vi "KE_scan_Gaussian_Fit.vi"(7 "NI DAQ (t) / Keithley (f)":bool, 8 "GaussFit der (f, def) / raw (t)":bool, 9 "Channel":i32=1 min=0 max=7 step=1, 10 "div I zero":bool=TRUE, 11 "KE scan Array":dbl[][](array[numeric])) -> (0 "error out":errorcluster, 1 "center":dbl format="%.1f", 2 "FWHM":dbl format="%.1f", 3 "KE scan Array OUT":dbl[][](array[numeric]), 4 "residue":dbl, 5 "XY Graph Array":cluster{dbl[], "Best Gaussian Fit":dbl[]}[](array[cluster]), 6 "offset":dbl)   [LabVIEW 2018]
uses:
  <vilib>/Analysis/6fits.llb/Curve Fitting Criteria.ctl
  <vilib>/Utility/file.llb/Read From Spreadsheet File (DBL).vi
  <vilib>/Analysis/NI_AALPro.lvlib
panel:
  out "XY Graph":T1(graph)
  in  "Density Factor (5)":dbl=5.0 format="%#_13g"
  out "Interpolated x-Axis":dbl[](array[numeric])
  in  "method (least square)":T2 items=["Least Square", "Least Absolute Residual", "Bisquare"]
  out "amplitude":dbl
  out "x-Axis":dbl[](array[numeric])
  out "abs(Derivative)":dbl[](array[numeric])
  out "Signal":dbl[](array[numeric])
  out "Best Gaussian Fit":dbl[](array[numeric])
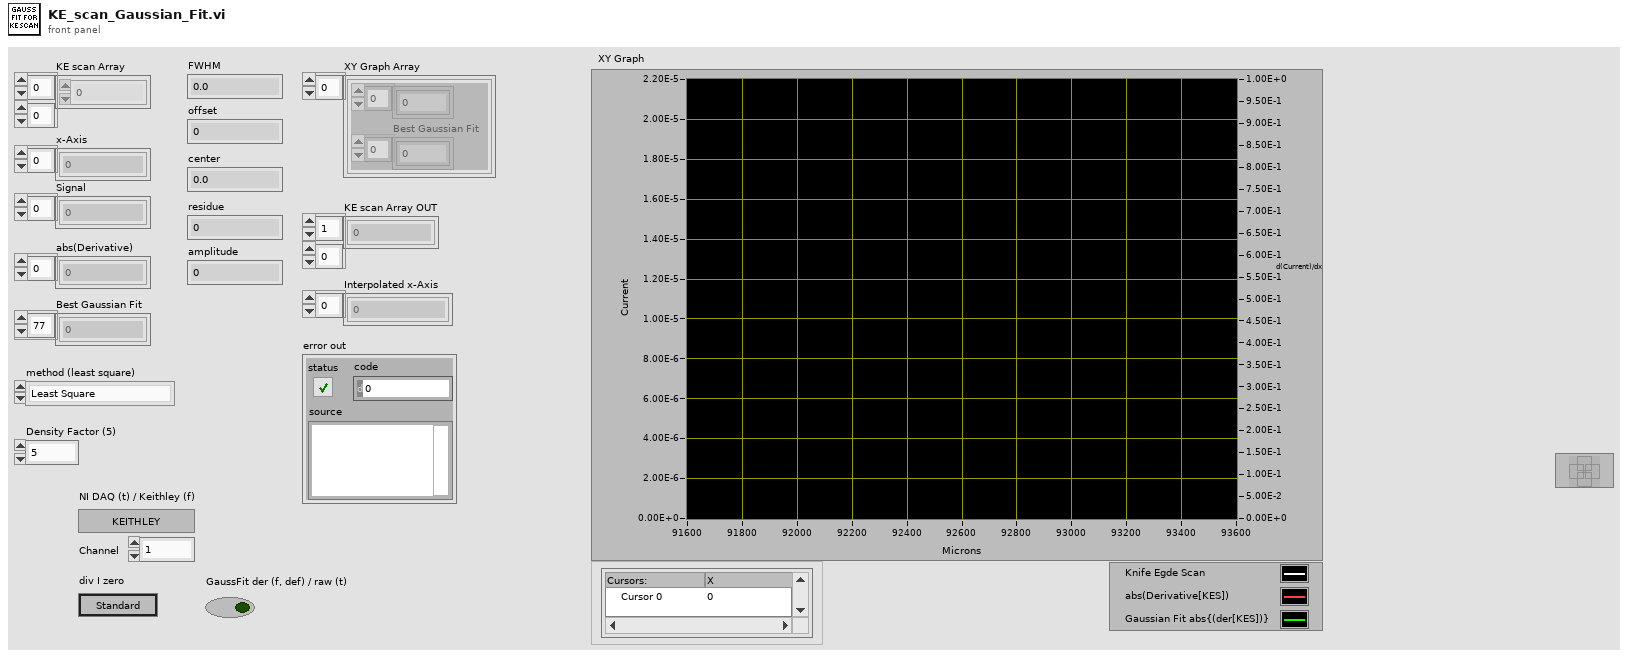
[diagram p1: front panel]
types:
  T1 = cluster{"Interpolated Array":dbl[], "Gaussian (Y)":dbl[]}[]
  T2 = typedef "NI_AALPro.lvlib/Curve Fitting Criteria.ctl" = u16
  T3 = cluster{"amp min":dbl, "amp max":dbl, "center min":dbl, "center max":dbl, "deviation min":dbl, "deviation max":dbl, "offset min":dbl, "offset max":dbl}
  T4 = cluster{"initial amplitude":dbl, "initial center":dbl, "initial standard deviation":dbl, "offset":dbl}
  T5 = cluster{"Interpolated Array":dbl[], "Gaussian (Y)":dbl[]}
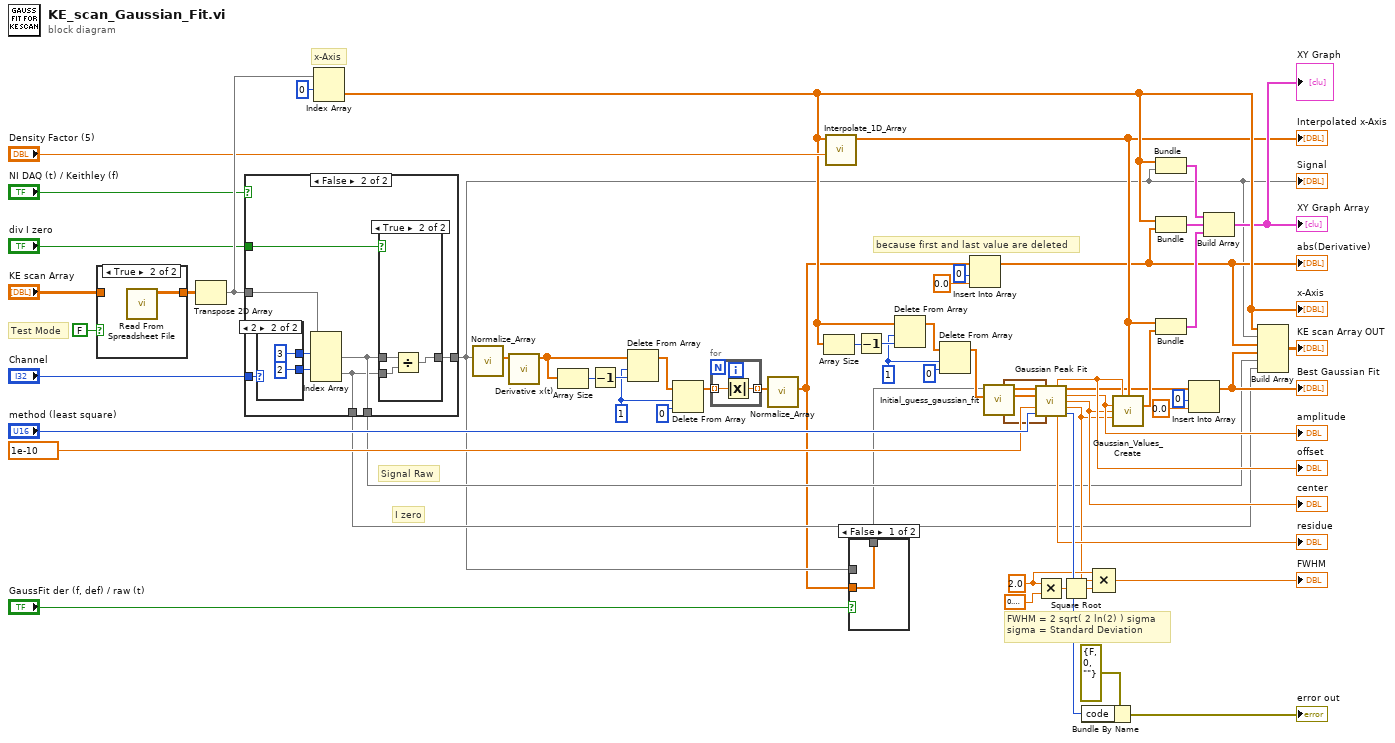
[diagram p0: block diagram]
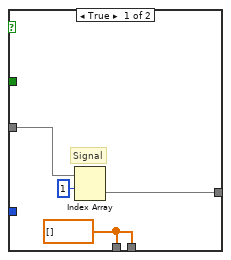
[diagram p3: hidden frame]
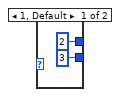
[diagram p5: hidden frame]
diagram:
  w40 = 1 ("length")
  w51 = 2.0 ("x")
  w59 = 1 ("length")
  # "I zero"
  # "Signal Raw"
  # "because first and last value are deleted"
  # "Test Mode"
  # "x-Axis"
  # "FWHM = 2 sqrt( 2 ln(2) ) sigma\nsigma = Standard Deviation"
  n1 = case shown="True" FALSE {
    tunnel: "KE scan Array" -> [w65 _]
    tunnel: [w65 w66] -> w27
    frame False {
    }
    frame True {
      n2 = call-poly <vilib>:"Read From Spreadsheet File.vi"() -> ("all rows"=w66:dbl[][])  [unwired: 7 in, 4 out]
    }
  }
  n3 = Transpose 2D Array(2D array=w27) -> (transposed array=w63:dbl[][])
  n4 = case shown="False" "NI DAQ (t) / Keithley (f)" {
    tunnel: w63 -> [w69 w77]
    tunnel: [w68 w74] -> w4
    tunnel: "Channel" -> [_ w75]
    tunnel: "div I zero" -> [_ w73]
    tunnel: [w67 w72] -> w6
    tunnel: [w67 w71] -> w5
    frame True {
      w67 = dbl[] []
      # "Signal"
      n5 = Index Array(array=w69, index (row)=1) -> (element=w68:dbl[])  [unwired: 1 in]
    }
    frame False {
      n6 = case shown="2" w75 {
        tunnel: [2 ("index (row)") 3 ("index (row)")] -> w78
        tunnel: [3 ("index (row)") 2 ("index (row)")] -> w76
        frame 1, Default {
        }
        frame 2 {
        }
      }
      n7 = Index Array(array=w77, index (row) #1=w78, index (row) #2=w76) -> (element #1=w72:dbl[], element #2=w71:dbl[])  [unwired: 2 in]
      n8 = case shown="True" w73 {
        tunnel: w72 -> [w79 w82]
        tunnel: w71 -> [_ w81]
        tunnel: [w79 w80] -> w74
        frame False {
        }
        frame True {
          n9 = Divide(x=w82, y=w81) -> (x/y=w80:dbl[])
        }
      }
    }
  }
  "Signal" <- w4
  n10 = Index Array(array=w63, index (row)=0) -> (element=w24:dbl[])  [unwired: 1 in]
  "x-Axis" <- w24
  n11 = call "Normalize_Array.vi"("array"=w4) -> ("normalized array"=w34:dbl[])  [unwired: 10 in]
  n12 = call <vilib>:"Derivative x(t).vi"("X"=w34) -> ("dX/dt"=w47:dbl[])  [unwired: 9 in, 1 out]
  n13 = Array Size(array=w47) -> (size(s)=w62:i32)
  n14 = Decrement(x=w62) -> (x-1=w61:i32)
  n15 = Delete From Array(array=w47, length=w59, index=w61) -> (array with subset deleted=w60:dbl[])  [unwired: 1 out]
  n16 = Delete From Array(array=w60, length=w59, index=0) -> (array with subset deleted=w57:dbl[])  [unwired: 1 out]
  n17 = for {
    tunnel: w57 -> [w88] mode=indexing
    tunnel: [w87] -> w31 mode=indexing
    n18 = Absolute Value(x=w88) -> (abs(x)=w87:dbl)
  }
  n19 = call "Normalize_Array.vi"("array"=w31) -> ("normalized array"=w3:dbl[])  [unwired: 10 in]
  n20 = Array Size(array=w24) -> (size(s)=w43:i32)
  n21 = call "Interpolate_1D_Array.vi"("Density Factor"="Density Factor (5)", "x-Axis in"=w24) -> ("Interpolated Array"=w17:dbl[])  [unwired: 9 in]
  "Interpolated x-Axis" <- w17
  n22 = case shown="False" "GaussFit der (f, def) / raw (t)" {
    tunnel: w4 -> [_ w90]
    tunnel: w3 -> [w89 _]
    tunnel: [w89 w90] -> w2
    frame False {
    }
    frame True {
    }
  }
  n23 = Decrement(x=w43) -> (x-1=w42:i32)
  n24 = Delete From Array(array=w24, length=w40, index=w42) -> (array with subset deleted=w41:dbl[])  [unwired: 1 out]
  n25 = Delete From Array(array=w41, length=w40, index=0) -> (array with subset deleted=w46:dbl[])  [unwired: 1 out]
  n26 = Insert Into Array(array=w3, index=0, new element=0.0 ("new element/subarray")) -> (w15:dbl[])
  "abs(Derivative)" <- w15
  n27 = call "Initial_guess_gaussian_fit.vi"("x-Axis in"=w46, "Signal in"=w2) -> ("x-Axis out"=w45:dbl[], "Signal out"=w44:dbl[], "Parameter Bounds Cluster"=w26:T3, "Initial Guess Cluster"=w32:T4)  [unwired: 2 in, 4 out]
  n28 = call <vilib>:"Gaussian Peak Fit.vi"("Y"=w44, "initial guess"=w32, "X"=w45, "tolerance"=1e-10, "method"="method (least square)", "parameter bounds"=w26) -> ("offset"=w23:dbl, "Best Gaussian Fit"=w11:dbl[], "amplitude"=w22:dbl, "center"=w21:dbl, "standard deviation"=w20:dbl, "residue"=→"residue":dbl, "error"=w55:i32)  [unwired: 3 in]
  "center" <- w21
  "offset" <- w23
  "amplitude" <- w22
  n29 = Multiply(x=w51, y=0.6931471805599453) -> (x*y=w52:dbl)
  n30 = Square Root(x=w52) -> (sqrt(x)=w50:dbl)
  n31 = Bundle By Name(cluster=errorcluster {"status"=FALSE, "code"=0, "source"=""} ("error in"), "code"=w55) -> (→"error out":errorcluster)
  n32 = Compound Arithmetic op=MULTIPLY(w51, w20, w50) -> (→"FWHM":dbl)
  n33 = call "Gaussian_Values_Create.vi"("offset"=w23, "X-Axis"=w17, "amplitude"=w22, "center"=w21, "sigma"=w20) -> ("Gaussian (Y)"=w18:dbl[])  [unwired: 10 in]
  n34 = Bundle(w24, w4) -> (w38:cluster{dbl[], dbl[]})  [unwired: 1 in]
  n35 = Bundle(w24, "normalized array"=w15) -> (w37:cluster{dbl[], "normalized array":dbl[]})  [unwired: 1 in]
  n36 = Bundle("Interpolated Array"=w17, "Gaussian (Y)"=w18) -> (w36:T5)  [unwired: 1 in]
  n37 = Insert Into Array(array=w11, index=0, new element=0.0 ("new element/subarray")) -> (w10:dbl[])
  "Best Gaussian Fit" <- w10
  n38 = Build Array(w38, w37, w36) -> (→"XY Graph Array" →"XY Graph":T1)
  n39 = Build Array(w24, w4, w15, w10, w6, w5) -> (→"KE scan Array OUT":dbl[][])
